vi "例题7.1.vi"() -> ()   [LabVIEW 2017]
panel:
  out "7（X0=10,dx=2,Y）多条曲线":cluster{i32, i32, cluster{dbl[]}[]}(graph)
  out "6（X0=10,dx=2,Y）多条曲线":cluster{i32, i32, dbl[][]}(graph)
  out "5（X0=10,dx=2,Y）多条曲线":cluster{i32, i32, dbl[]}[](graph)
  out "4（X0=10,dx=2,Y）单条曲线":cluster{i32, i32, dbl[]}(graph)
  out "3（Y）多条曲线":cluster{dbl[]}[](graph)
  out "2（Y）多条曲线":dbl[][](graph)
  out "1（Y）单条曲线":dbl[](graph)
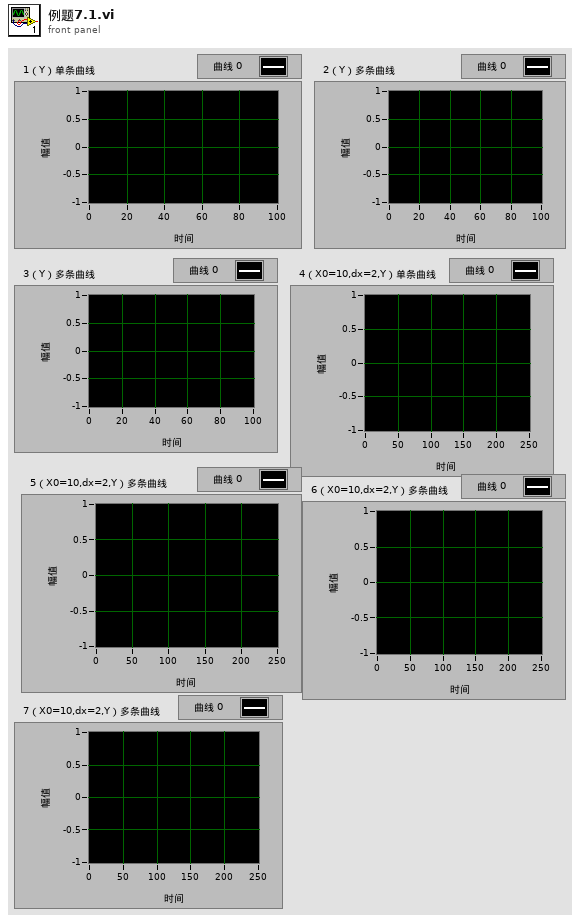
[diagram p1: front panel]
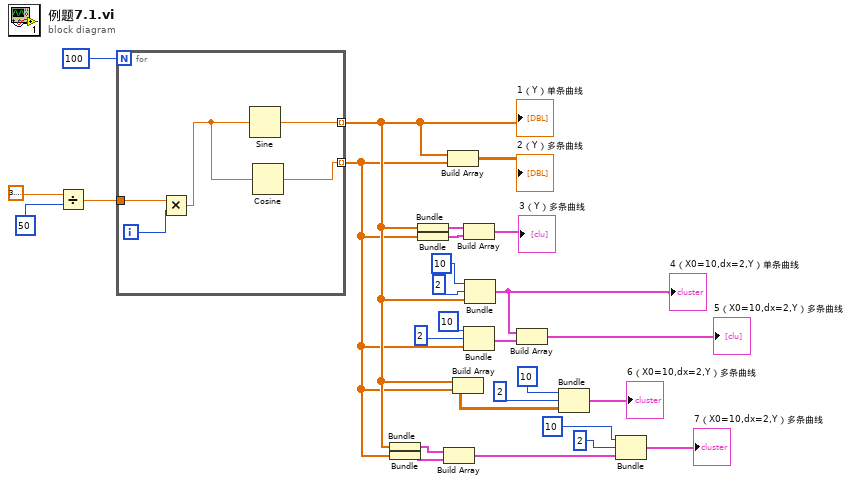
[diagram p0: block diagram]
diagram:
  n1 = Divide(x=3.141592653589793, y=50) -> (x/y=w26:dbl)
  n2 = for {
    N: 100 -> [_]
    tunnel: w26 -> [w32]
    tunnel: [w29] -> w4 mode=indexing
    tunnel: [w28] -> w3 mode=indexing
    i -> [w30]
    n3 = Multiply(x=w32, y=w30) -> (x*y=w31:dbl)
    n4 = Sine(x=w31) -> (sin(x)=w29:dbl)
    n5 = Cosine(x=w31) -> (cos(x)=w28:dbl)
  }
  "1（Y）单条曲线" <- w4
  n6 = Bundle(w4) -> (w17:cluster{dbl[]})  [unwired: 1 in]
  n7 = Bundle(w3) -> (w1:cluster{dbl[]})  [unwired: 1 in]
  n8 = Bundle(w4) -> (w2:cluster{dbl[]})  [unwired: 1 in]
  n9 = Bundle(w3) -> (w24:cluster{dbl[]})  [unwired: 1 in]
  n10 = Build Array(w17, w1) -> (w16:cluster{dbl[]}[])
  n11 = Build Array(w4, w3) -> (→"2（Y）多条曲线":dbl[][])
  n12 = Build Array(w4, w3) -> (w18:dbl[][])
  n13 = Build Array(w2, w24) -> (→"3（Y）多条曲线":cluster{dbl[]}[])
  n14 = Bundle(10, 2, w3) -> (w20:cluster{i32, i32, dbl[]})  [unwired: 1 in]
  n15 = Bundle(10, 2, w4) -> (w9:cluster{i32, i32, dbl[]})  [unwired: 1 in]
  "4（X0=10,dx=2,Y）单条曲线" <- w9
  n16 = Build Array(w9, w20) -> (→"5（X0=10,dx=2,Y）多条曲线":cluster{i32, i32, dbl[]}[])
  n17 = Bundle(10, 2, w18) -> (→"6（X0=10,dx=2,Y）多条曲线":cluster{i32, i32, dbl[][]})  [unwired: 1 in]
  n18 = Bundle(10, 2, w16) -> (→"7（X0=10,dx=2,Y）多条曲线":cluster{i32, i32, cluster{dbl[]}[]})  [unwired: 1 in]
